vi "set_calibration.vi"(8 "error in (no error)":errorcluster, 10 "calibration":T1, 11 "GenericTrajectory.lvclass in":refnum<class "TrajectoryDL091126GenericVoxel.lvclass">) -> (0 "error out":errorcluster, 3 "GenericTrajectory.lvclass out":refnum<class "TrajectoryDL091126GenericVoxel.lvclass">)   [LabVIEW 2010, in "TrajectoryDL091126GenericVoxel.lvclass"]
uses:
  TrajectoryDL091126GenericVoxel.lvclass
  common/clusters/calibration.ctl
  common/enumerations/unit.ctl
  TrajectoryDL091126GenericVoxel.lvclass/TrajectoryDL091126GenericVoxel.ctl
  common/classes/Image/Image/Image.lvclass
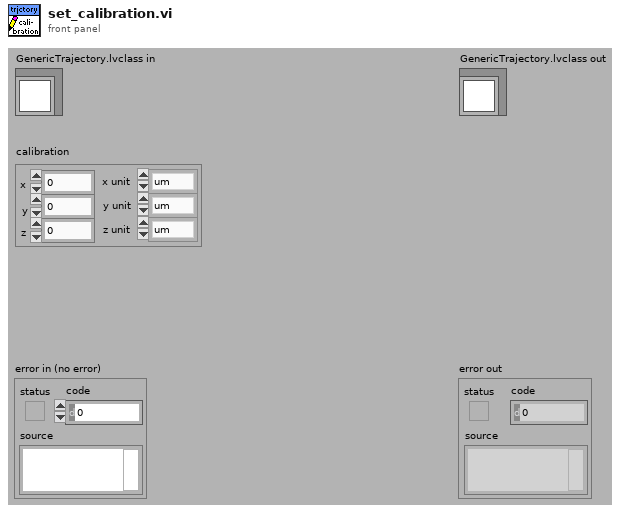
[diagram p1: front panel]
types:
  T1 = typedef "calibration.ctl" = cluster{"x":dbl, "y":dbl, "z":dbl, "x unit":T2, "y unit":T2, "z unit":T2}
  T2 = typedef "Image.lvclass/unit.ctl" = enum16{"um", "s"}
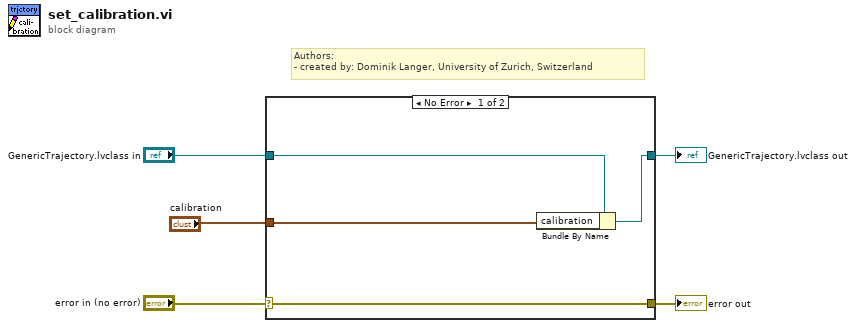
[diagram p0: block diagram]
diagram:
  # "Authors: \n- created by: Dominik Langer, University of Zurich, Switzerland"
  n1 = case shown="No Error" "error in (no error)" {
    selector: "error in (no error)" -> [w9 w10]
    tunnel: [w9 w10] -> w4
    tunnel: [w7 w11] -> w2
    tunnel: "GenericTrajectory.lvclass in" -> [w8 w11]
    tunnel: "calibration" -> [w6 _]
    frame No Error {
      n2 = Bundle By Name(cluster=w8, "calibration"=w6) -> (w7:refnum<class "TrajectoryDL091126GenericVoxel.lvclass">)
    }
    frame Error {
    }
  }
  "error out" <- w4
  "GenericTrajectory.lvclass out" <- w2
